vi "Config Reference Mode.vi"(8 "error in":errorcluster, 10 "Reference Mode (on)":enum16{"off", "on"}(ring)=enum."on", 11 "VISA resource name":refnum<visa-resource-name>) -> (0 "error out":errorcluster, 3 "VISA resource name out":refnum<visa-resource-name>)   [LabVIEW 2019, in "Andeen-Hagerling 2700(400 firmware).lvlib"]
doc: "Reference result mode is enabled when set to ON."
uses:
  Andeen-Hagerling 2700(400 firmware).lvlib
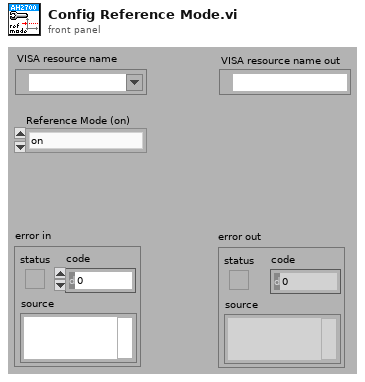
[diagram p1: front panel]
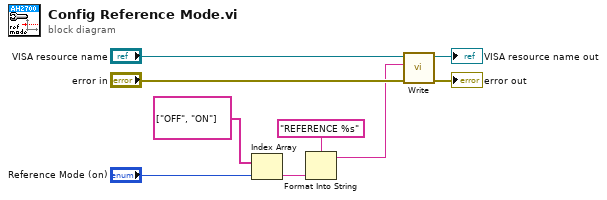
[diagram p0: block diagram]
diagram:
  n1 = Index Array(array=string[] ["OFF", "ON"], index="Reference Mode (on)") -> (element=w1:string)
  n2 = Format Into String(format string="REFERENCE %s", w1) -> (resulting string=w4:string)  [unwired: 2 in, 1 out]
  n3 = call "Write.vi"("error in"="error in", "command"=w4, "VISA resource name"="VISA resource name") -> ("error out"=→"error out":errorcluster, "VISA resource name out"=→"VISA resource name out":refnum<visa-resource-name>)  [unwired: 7 in]
